vi "Tag-FPGA-))Channel-NoOp.vi"(8 "abort (F)":bool, 10 "element in":cluster{timestamp[], dbl[]}[](array[cluster]), 11 "channelOp":T1) -> (0 "aborted?":bool, 2 "element out":i32, 3 "sequence":i16)   [LabVIEW 2020, in "Tag-a[.](c(a[.](stamp),a[.](dbl))).lvlib"]
uses:
  <extravilib>/ChannelInstances/Tag-a[.](c(a[.](stamp),a[.](dbl))).lvlib
  <extravilib>/ChannelInstances/Tag-a[.](c(a[.](stamp),a[.](dbl)))/ChannelOp.ctl
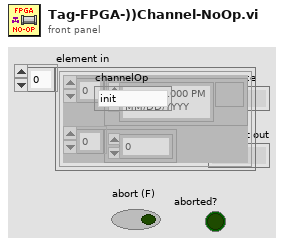
[diagram p1: front panel]
types:
  T1 = typedef "Tag-a[.](c(a[.](stamp),a[.](dbl))).lvlib/ChannelOp.ctl" = enum16{"init", "write", "read", "probe"}
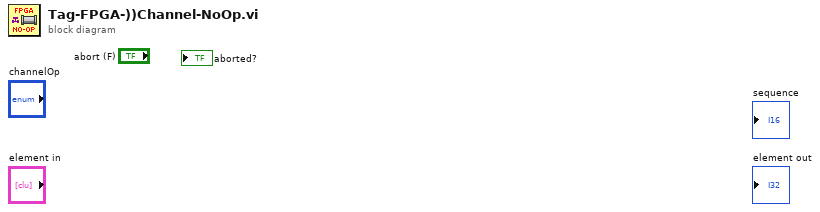
[diagram p0: block diagram]
diagram:
